vi "WPI_GyroXRS450_SPI_GetSet_Data.vi"(0 "GyroDeviceRef":T1={"DevStatus"={"status"=FALSE, "code"=0, "source"=""}, "Analog Channel"=enum."AI 0", "Gain (VoltsPerDegree/Second)"=0.0, "Gyro Type"=enum."Analog", "Handle"=0, "SPI Bus"=enum."Invalid", "Device Found"=FALSE, "Sample Rate"=1.0, "Calibrate On Open"=FALSE, "Offset"=0.0} {"Sample Rate" min=0.25 max=100.0 step=0.25}, 1 "Operation":enum16{"set", "get"}(ring), 5 "Offset":dbl, 7 "Calibrated":bool, 9 "Angle":dbl, 11 "Rate":dbl) -> (4 "GyroDeviceRef":T1={"DevStatus"={"status"=FALSE, "code"=0, "source"=""}, "Analog Channel"=enum."AI 0", "Gain (VoltsPerDegree/Second)"=0.0, "Gyro Type"=enum."Analog", "Handle"=0, "SPI Bus"=enum."Invalid", "Device Found"=FALSE, "Sample Rate"=1.0, "Calibrate On Open"=FALSE, "Offset"=0.0} {"Sample Rate" min=0.25 max=100.0 step=0.25}, 6 "Offset":dbl, 8 "Calibrated?":bool, 10 "Angle":dbl, 15 "Rate":dbl)   [LabVIEW 2017]
uses:
  <vilib>/Rock Robotics/WPI/Gyro/WPI_GyroDevRef.ctl
  <vilib>/Rock Robotics/SystemInterfaces/AI/FPGA_AIChannel.ctl
  <vilib>/Rock Robotics/SystemInterfaces/spilib/spi_bus.ctl
panel:
  # "Analog"
  # "XRS"
  # "Analog"
  # "XRS"
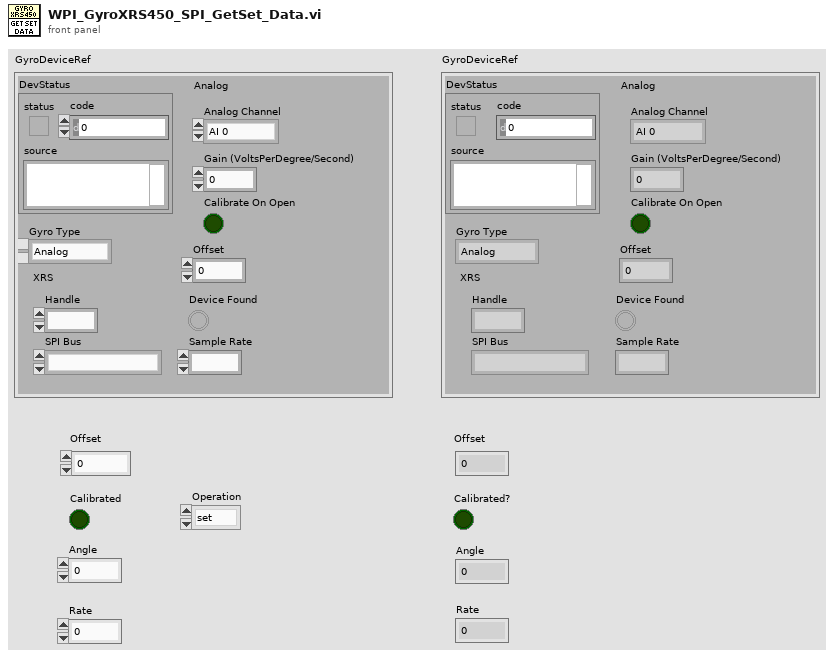
[diagram p1: front panel]
types:
  T1 = typedef "WPI_GyroDevRef.ctl" = cluster{"DevStatus":errorcluster, "Analog Channel":T2, "Gain (VoltsPerDegree/Second)":dbl, "Gyro Type":enum16{"Analog", "XRS450"}, "Handle":i32, "SPI Bus":T3, "Device Found":bool, "Sample Rate":dbl, "Calibrate On Open":bool, "Offset":dbl}
  T2 = typedef "FPGA_AIChannel.ctl" = enum8{"AI 0", "AI 1", "AI 2", "AI 3", "AI MXP 0", "AI MXP 1", "AI MXP 2", "AI MXP 3", "Invalid"}
  T3 = typedef "spi_bus.ctl" = enum16{"SPI On-Board, CS0", "SPI On-Board, CS1", "SPI On-Board, CS2", "SPI On-Board, CS3", "SPI MXP", "Invalid"}
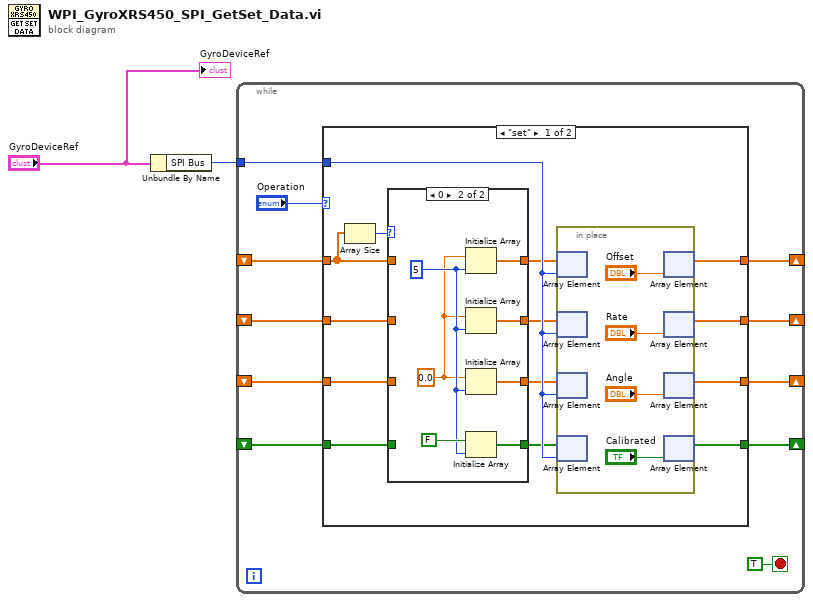
[diagram p0: block diagram]
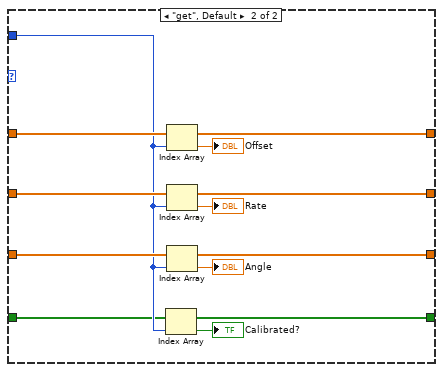
[diagram p3: hidden frame]
diagram:
  n1 = Unbundle By Name("GyroDeviceRef") -> ("SPI Bus"=w2:T3)
  n2 = while {
    tunnel: w2 -> [w7]
    shift-right: [w11] -> _
    shift-left: _ -> [w9]
    shift-right: [w10] -> _
    shift-left: _ -> [w8]
    shift-right: [w6] -> _
    shift-left: _ -> [w5]
    shift-right: [w4] -> _
    shift-left: _ -> [w3]
    stop <- TRUE stop-if-true
    n3 = case shown="\"set\"" "Operation" {
      tunnel: [w21 w51] -> w11
      tunnel: [w20 w50] -> w10
      tunnel: w9 -> [w26 w51]
      tunnel: w8 -> [w25 w50]
      tunnel: w7 -> [w24 w44]
      tunnel: [w19 w47] -> w6
      tunnel: w5 -> [w23 w47]
      tunnel: [w18 w43] -> w4
      tunnel: w3 -> [w22 w43]
      frame "set" {
        n4 = Array Size(array=w26) -> (size(s)=w27:i32)
        n5 = case shown="0" w27 {
          tunnel: [w35 w42] -> w17
          tunnel: [w33 w41] -> w15
          tunnel: w26 -> [w35 _]
          tunnel: w25 -> [w33 _]
          tunnel: [w34 w40] -> w16
          tunnel: w23 -> [w34 _]
          tunnel: [w32 w37] -> w14
          tunnel: w22 -> [w32 _]
          frame 5, Default {
          }
          frame 0 {
            w36 = 0.0 ("Angle")
            w38 = 5 ("dimension size")
            n6 = Initialize Array(w36, w38) -> (w42:dbl[])
            n7 = Initialize Array(w36, w38) -> (w40:dbl[])
            n8 = Initialize Array(w36, w38) -> (w41:dbl[])
            n9 = Initialize Array(FALSE, w38) -> (w37:bool[])
          }
        }
        n10 = in-place {
          n11 = in-place-array #1(w17, w24) -> ()  [unwired: 1 out]
          n12 = in-place-array #2(w16, w24) -> ()  [unwired: 1 out]
          n13 = in-place-array #3(w15, w24) -> ()  [unwired: 1 out]
          n14 = in-place-array #4(w14, w24) -> ()  [unwired: 1 out]
          n15 = in-place-array #1("Offset") -> (w21:dbl[])  [unwired: 1 out]
          n16 = in-place-array #2("Rate") -> (w19:dbl[])  [unwired: 1 out]
          n17 = in-place-array #3("Angle") -> (w20:dbl[])  [unwired: 1 out]
          n18 = in-place-array #4("Calibrated") -> (w18:bool[])  [unwired: 1 out]
        }
      }
      frame "get", Default {
        n19 = Index Array(array=w43, index=w44) -> (element=→"Calibrated?":bool)
        n20 = Index Array(array=w51, index=w44) -> (element=→"Offset":dbl)
        n21 = Index Array(array=w47, index=w44) -> (element=→"Rate":dbl)
        n22 = Index Array(array=w50, index=w44) -> (element=→"Angle":dbl)
      }
    }
  }
  "GyroDeviceRef" <- "GyroDeviceRef"
